vi "BMP初始化.vi"() -> (3 "簇":T1)   [LabVIEW 2012]
panel:
  in  "path to BMP file":path=path "D:/project/MyVI/扫雷/icons.bmp" caption="BMP文件路径"
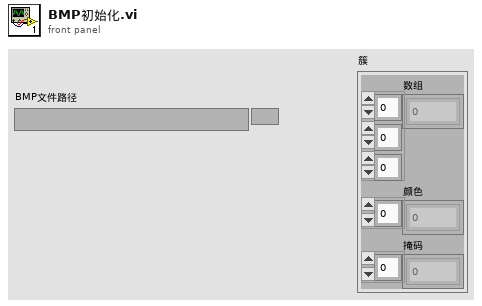
[diagram p1: front panel]
types:
  T1 = cluster{"数组":i32[][][], "colors":u32[], "mask":u8[]}
  T2 = typedef "imagedata.ctl" = cluster{"image type":i32, "image depth":i32, "image":u8[], "mask":u8[], "colors":u32[], "Rectangle":cluster{"left":i16, "top":i16, "right":i16, "bottom":i16}}
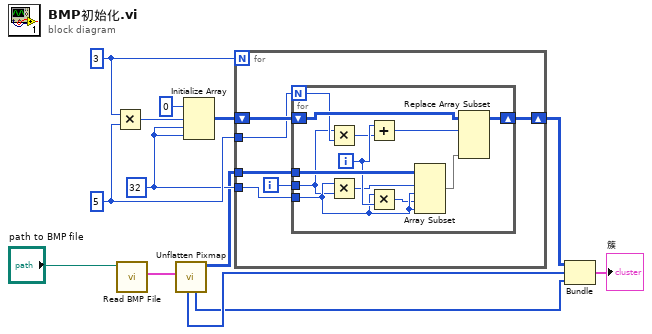
[diagram p0: block diagram]
diagram:
  w6 = 32
  w8 = 5
  w9 = 3
  n1 = Multiply(x=w9, y=w8) -> (x*y=w7:i32)
  n2 = call <vilib>:"Read BMP File.vi"("path to BMP file"="path to BMP file") -> ("image data"=w12:T2)  [unwired: 8 in, 2 out]
  n3 = call <vilib>:"Unflatten Pixmap.vi"("image data"=w12) -> ("24-bit pixmap"=w5:u32[][], "colors"=w1:u32[], "mask"=w2:u8[])  [unwired: 4 in, 4 out]
  n4 = Initialize Array(0, w7, w6, w6) -> (w10:i32[][][])
  n5 = for {
    N: w9 -> [_]
    tunnel: w5 -> [w19]
    tunnel: w8 -> [w17]
    tunnel: w6 -> [w16]
    shift-right: [w15] -> w3
    shift-left: w10 -> [w18]
    i -> [w14]
    n6 = for {
      N: w17 -> [w23]
      tunnel: w19 -> [w29]
      tunnel: w14 -> [w20]
      tunnel: w16 -> [w27]
      shift-right: [w26] -> w15
      shift-left: w18 -> [w31]
      i -> [w28]
      n7 = Multiply(x=w20, y=w23) -> (x*y=w21:i32)
      n8 = Multiply(x=w27, y=w20) -> (x*y=w24:i32)
      n9 = Add(x=w28, y=w21) -> (x+y=w30:i32)
      n10 = Multiply(x=w27, y=w28) -> (x*y=w25:i32)
      n11 = Array Subset(array=w29, index (row)=w24, length (row)=w27, index (col)=w25, length (col)=w27) -> (w22:u32[][])
      n12 = Replace Array Subset(array=w31, new element=w22, index (dim 0)=w30) -> (w26:i32[][][])  [unwired: 2 in]
    }
  }
  n13 = Bundle(w3, "mask"=w2, "colors"=w1) -> (→"簇":cluster{i32[][][], "mask":u8[], "colors":u32[]})  [unwired: 1 in]
